vi "Set Host to Target DMAMapvi.vi"(8 "error in (no error)":errorcluster, 10 "DMA configuration array":T1[](array[typedef])=[{"Name"="P2PSource", "Depth"=1023, "Write? (Deprecated:Use Implementation)"=TRUE, "Physical Channel"=0, "Base Address"=65472, "Data Width"=32, "Data Type"=enum."U32", "FXP Properties"=variant(fxp<+,32,32> 0.0), "Write Window Address"=0, "Implementation"=enum."niFpgaPeerToPeerWriter", "Control Set"=0}, {"Name"="P2PSink", "Depth"=1023, "Write? (Deprecated:Use Implementation)"=FALSE, "Physical Channel"=1, "Base Address"=65408, "Data Width"=32, "Data Type"=enum."U32", "FXP Properties"=variant(fxp<+,32,32> 0.0), "Write Window Address"=57344, "Implementation"=enum."niFpgaPeerToPeerReader", "Control Set"=1}], 11 "Item Ref in":T4 format="%.0x") -> (0 "error out":errorcluster, 3 "Item Ref out":T4 format="%.0x")   [LabVIEW 2016]
uses:
  <vilib>/NI VeriStand/Custom Device API/Custom Device API.lvlib
  Shared/Constants.vi
  Shared/FPGA Addon Shared.lvlib
  <vilib>/NI VeriStand/Custom Device Tools/Custom Device Utility Library/Custom Device Utility Library.lvlib
  <vilib>/NI Veristand/Custom Device API/Custom Device Item Ref.ctl
  <vilib>/NI Veristand/Custom Device API/Set Item Property (Variant).vi
  <vilib>/rvi/DataTransferAndStorage/Container/Common/niFpgaDataTypeControl.ctl
  <vilib>/rvi/ClientSDK/Core/ModuleGeneration/CommunicationInterfaceUtility/niFpgaDmaChannelImplementation.ctl
  <vilib>/rvi/FIFO/Fifo_Types/Fifo_DMA_Config.ctl
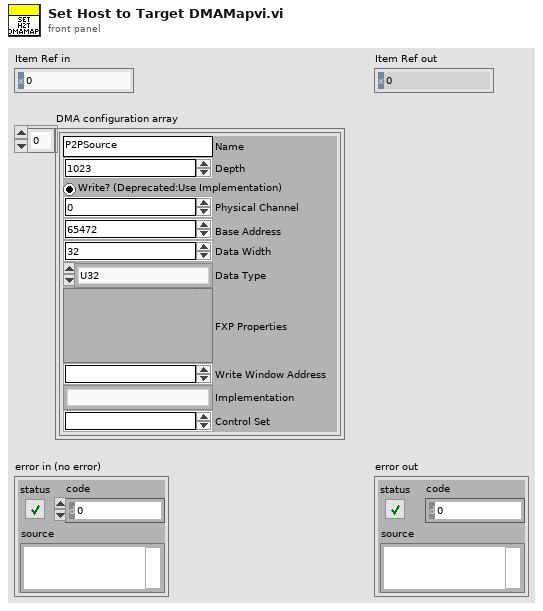
[diagram p1: front panel]
types:
  T1 = typedef "Fifo_DMA_Config.ctl" = cluster{"Name":string, "Depth":u32, "Write? (Deprecated:Use Implementation)":bool, "Physical Channel":u32, "Base Address":u32, "Data Width":u32, "Data Type":T2, "FXP Properties":variant, "Write Window Address":u32, "Implementation":T3, "Control Set":u32}
  T2 = typedef "niFpgaDataTypeControl.ctl" = enum32{"Boolean", "I8", "I16", "I32", "I64", "U8", "U16", "U32", "U64", "FXP", "CustomControl", "SGL"}
  T3 = typedef "niFpgaDmaChannelImplementation.ctl" = enum16{"niFpgaTargetToHost", "niFpgaHostToTarget", "niFpgaPeerToPeerWriter", "niFpgaPeerToPeerReader", "niCoreTargetToHost", "niCoreHostToTarget"}
  T4 = typedef "Custom Device API.lvlib/Custom Device Item Ref.ctl" = u64
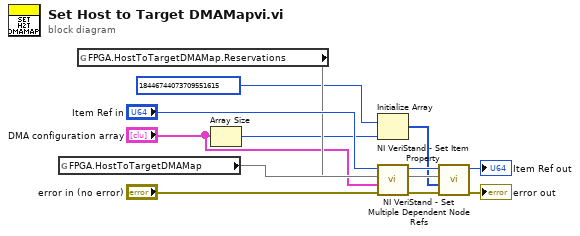
[diagram p0: block diagram]
diagram:
  n1 = global read "Constants.vi" "FPGA.HostToTargetDMAMap"() -> (w10)
  n2 = global read "Constants.vi" "FPGA.HostToTargetDMAMap.Reservations"() -> (w5)
  n3 = Array Size(array="DMA configuration array") -> (size(s)=w2:i32)
  n4 = Initialize Array(T4 18446744073709551615 ("Item Ref out"), w2) -> (w3:T4[])
  n5 = call-poly <vilib>:"NI VeriStand - Set Item Property.vi"("error in (no error)"="error in (no error)", "Value"="DMA configuration array", "Property Name"=w10, "Item Ref in"="Item Ref in") -> ("error out"=w12:errorcluster, "Item Ref out"=w7:T4)  [unwired: 5 in, 1 out]
  n6 = call <vilib>:"NI VeriStand - Set Multiple Dependent Node Refs.vi"("error in (no error)"=w12, "Dependent Node Refs"=w3, "Base Property Name"=w5, "Item Ref in"=w7) -> ("error out"=→"error out":errorcluster, "Item Ref out"=→"Item Ref out":T4)  [unwired: 6 in]
